vi "connect.vi"(6 "timeout ms (10000)":i32=10000, 8 "error in":errorcluster, 11 "TCP client in":refnum<class "TCP client.lvclass">) -> (0 "error out":errorcluster, 1 "valid?":bool, 2 "new connection":refnum<class "connection maintainer.lvclass">, 3 "TCP client out":refnum<class "TCP client.lvclass">)   [LabVIEW 2015, in "TCP client.lvclass"]
uses:
  TCP client.lvclass
  connection/connection maintainer.lvclass
  client/connection client.lvclass/connection client.ctl
  TCP connection/TCP connection.lvclass/TCP connection.ctl
  TCP connection/TCP connection.lvclass
  client/connection client.lvclass
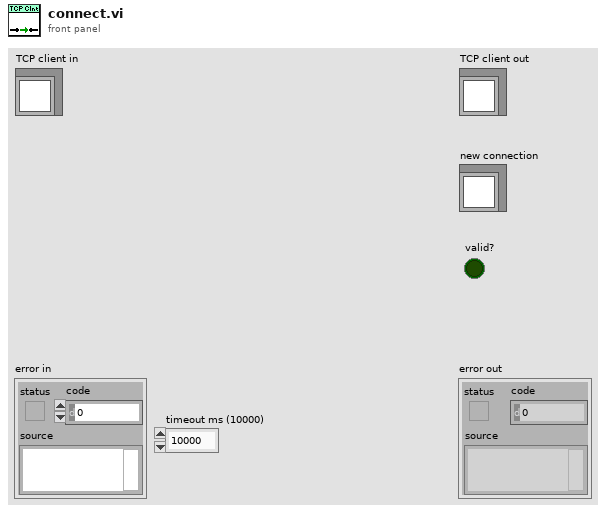
[diagram p1: front panel]
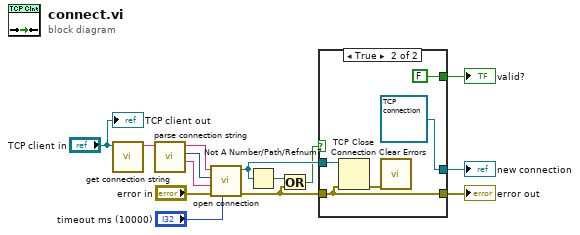
[diagram p0: block diagram]
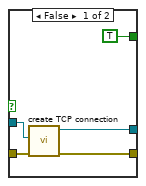
[diagram p2: hidden frame]
diagram:
  n1 = call "get connection string.vi"("connection client in"="TCP client in") -> ("connection string"=w14:string)  [unwired: 10 in]
  n2 = call "parse connection string.vi"("connection string in"=w14) -> ("service name"=w10:string, "port"=w11:u16, "address"=w12:string)  [unwired: 8 in]
  n3 = call "open connection.vi"("timeout ms (60000)"="timeout ms (10000)", "error in (no error)"="error in", "service name"=w10, "port"=w11, "address"=w12) -> ("error out"=w1:errorcluster, "TCP Network Connection out"=w4:refnum<k5>)  [unwired: 5 in]
  n4 = Not A Number/Path/Refnum?(number/path/refnum=w4) -> (NaN/Path/Refnum?=w7:bool)
  n5 = Or(x=w7, y=w1) -> (x .or. y?=w2:bool)
  n6 = case shown="True" w2 {
    tunnel: [TRUE FALSE] -> w6
    tunnel: [w17 w21] -> w5
    tunnel: w1 -> [w18 w21]
    tunnel: w4 -> [w16 w22]
    tunnel: [w15 refnum<class "TCP connection.lvclass"> refnum ("TCP connection out")] -> w3
    frame False {
      n7 = call "create TCP connection.vi"("error in"=w18, "connection"=w16) -> ("error out"=w17:errorcluster, "TCP connection out"=w15:refnum<class "TCP connection.lvclass">)  [unwired: 8 in]
    }
    frame True {
      n8 = TCP Close Connection(connection ID=w22, error in (no error)=w21) -> (error out=w20:errorcluster)  [unwired: 1 in, 1 out]
      n9 = call <vilib>:"Clear Errors.vi"("error in (no error)"=w20) -> ()  [unwired: 5 in, 2 out]
    }
  }
  "error out" <- w5
  "new connection" <- w3
  "valid?" <- w6
  "TCP client out" <- "TCP client in"
